vi "Limelight LED Control.vi"(0 "Auto-Align":bool) -> ()   [LabVIEW 2019]
uses:
  <vilib>/Rock Robotics/Network Tables/NT Write Number.vi
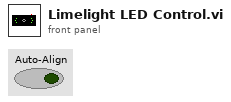
[diagram p1: front panel]
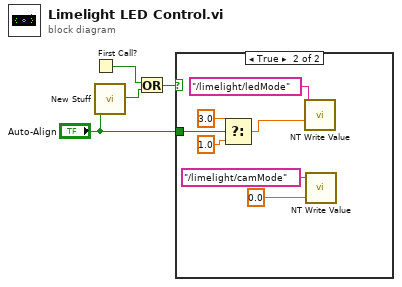
[diagram p0: block diagram]
diagram:
  n1 = First Call?() -> (First Call?: T/F=w2:bool)
  n2 = call "New Stuff.vi"("Variant 14"="Auto-Align") -> ("x != y?"=w3:bool)  [unwired: 26 in]
  n3 = Or(x=w2, y=w3) -> (x .or. y?=w1:bool)
  n4 = case shown="True" w1 {
    tunnel: "Auto-Align" -> [_ w7]
    frame False {
    }
    frame True {
      n5 = Select(t=3.0, s=w7, f=1.0) -> (s? t:f=w10:dbl)
      n6 = call-poly <vilib>:"NT Write Value.vi"("Numeric"=w10, "Name"="/limelight/ledMode") -> ()  [unwired: 9 in, 1 out]
      n7 = call-poly <vilib>:"NT Write Value.vi"("Numeric"=0.0, "Name"="/limelight/camMode") -> ()  [unwired: 9 in, 1 out]
    }
  }
